vi "Read Alarm Output.vi"(7 "Unit Address (1)":u8=1, 8 "error in (no error)":errorcluster, 9 "Enable Alarm Group (True)":bool=TRUE, 10 "Alarm Number (1)":u16=1 min=1 max=8, 11 "VISA resource name":refnum<visa-resource-name>) -> (0 "error out":errorcluster, 2 "Alarm Output":bool, 3 "VISA resource name out":refnum<visa-resource-name>)   [LabVIEW 2014, in "Eurotherm 35xx Series.lvlib"]
doc: "This VI reads Alarm output value."
uses:
  <instrlib>/Eurotherm 35xx Series/Eurotherm 35xx Series.lvlib
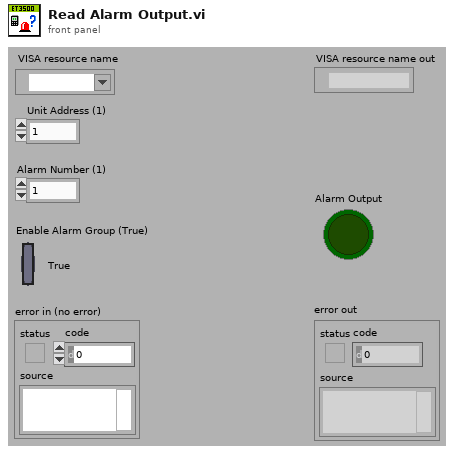
[diagram p1: front panel]
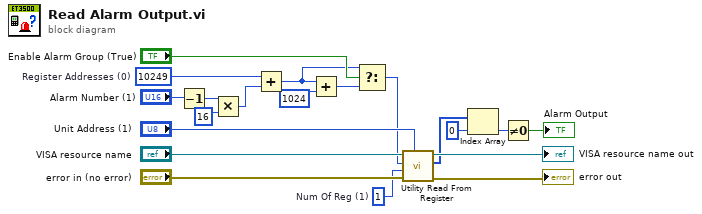
[diagram p0: block diagram]
diagram:
  w15 = u16 1  # Num Of Reg (1)
  w6 = 10249  # Register Addresses (0)
  n1 = Decrement(x="Alarm Number (1)") -> (x-1=w9:u16)
  n2 = Multiply(x=w9, y=u16 16) -> (x*y=w7:u16)
  n3 = Add(x=w6, y=w7) -> (x+y=w2:i32)
  n4 = Add(x=w2, y=1024) -> (x+y=w3:i32)
  n5 = Select(t=w2, s="Enable Alarm Group (True)", f=w3) -> (s? t:f=w1:i32)
  n6 = call <instrlib>:"Utility Read From Register.vi"("Unit Address (1)"="Unit Address (1)", "error in (no error)"="error in (no error)", "Num Of Reg (1)"=w15, "Register Address (0)"=w1, "VISA resource name"="VISA resource name") -> ("error out"=→"error out":errorcluster, "Data"=w14:i16[], "VISA resource name out"=→"VISA resource name out":refnum<visa-resource-name>)  [unwired: 4 in]
  n7 = Index Array(array=w14, index=0) -> (element=w12:i16)
  n8 = Not Equal To 0?(x=w12) -> (x != 0?=→"Alarm Output":bool)
